vi "Abort Multipart Upload.vi"(8 "error in (no error)":errorcluster, 11 "Multipart Upload RefNum in":T1) -> (0 "error out":errorcluster, 2 "No Such Upload":bool, 3 "Multipart Upload RefNum out":T1)   [LabVIEW 2011, in "LV Interface for Amazon S3.lvlib"]
doc: "This operation <B>aborts a multipart upload</B>. After a multipart upload is aborted, <B>no additional parts can be uploaded using that multipart upload reference</B>. The <B>storage consumed</B> by any previously uploaded parts <B>will be freed</B>. However, <B>if any part uploads are currently in progress, those</B> part uploads <B>might or might not succeed</B>. As a result, <B>it might be necessary to abort a given multipart upload multiple times</B> in order to completely free all storage consumed by all parts."
uses:
  LV Interface for Amazon S3.lvlib
  Typedefs/AMZ_S3_Multipart Upload RefNum.ctl
  Typedefs/AMZ_S3_Multipart Upload RefNum Enum.ctl
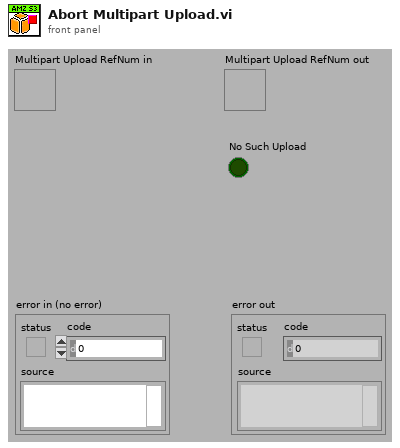
[diagram p1: front panel]
types:
  T1 = typedef "LV Interface for Amazon S3.lvlib/AMZ_S3_Multipart Upload RefNum.ctl" = refnum<k1>
  T2 = typedef "LV Interface for Amazon S3.lvlib/AMZ_S3_Multipart Upload Data.ctl" = cluster{"Object":string, "Bucket":string, "UploadID":string, "Parts":T3[]}
  T3 = typedef "LV Interface for Amazon S3.lvlib/AMZ_S3_Multipart Upload Part Data.ctl" = cluster{"PartNumber":u16, "Lat modified":timestamp, "ETag":string, "Size":u64}
  T4 = typedef "LV Interface for Amazon S3.lvlib/AMZ_S3_Call Results.ctl" = enum16{"Success", "UndefinedError", "AccessDenied", "AccountProblem", "AmbiguousGrantByEmailAddress", "BadDigest", "BucketAlreadyExists", "BucketAlreadyOwnedByYou", "BucketNotEmpty", "CredentialsNotSupported", "CrossLocationLoggingProhibited", "EntityTooSmall", "EntityTooLarge", "ExpiredToken", "IllegalVersioningConfigurationException", "IncompleteBody", "IncorrectNumberOfFilesInPostRequest", "InlineDataTooLarge", "InternalError", "InvalidAccessKeyId", "InvalidAddressingHeader", "InvalidArgument", "InvalidBucketName", "InvalidDigest", "InvalidLocationConstraint", "InvalidPart", "InvalidPartOrder", "InvalidPayer", "InvalidPolicyDocument", "InvalidRange", "InvalidSecurity", "InvalidSOAPRequest", "InvalidStorageClass", "InvalidTargetBucketForLogging", "InvalidToken", "InvalidURI", "KeyTooLong", "MalformedACLError", "MalformedPOSTRequest", "MalformedXML", "MaxMessageLengthExceeded", "MaxPostPreDataLengthExceededError", "MetadataTooLarge", "MethodNotAllowed", "MissingAttachment", "MissingContentLength", "MissingRequestBodyError", "MissingSecurityElement", "MissingSecurityHeader", "NoLoggingStatusForKey", "NoSuchBucket", "NoSuchKey", "NoSuchUpload", "NoSuchVersion", "NotImplemented", "NotSignedUp", "OperationAborted", "PermanentRedirect", "PreconditionFailed", "Redirect", "RequestIsNotMultiPartContent", "RequestTimeout", "RequestTimeTooSkewed", "RequestTorrentOfBucketError", "SignatureDoesNotMatch", "SlowDown", "TemporaryRedirect", "TokenRefreshRequired", "TooManyBuckets", "UnexpectedContent", "UnresolvableGrantByEmailAddress", "UserKeyMustBeSpecified", "LabVIEWError"}
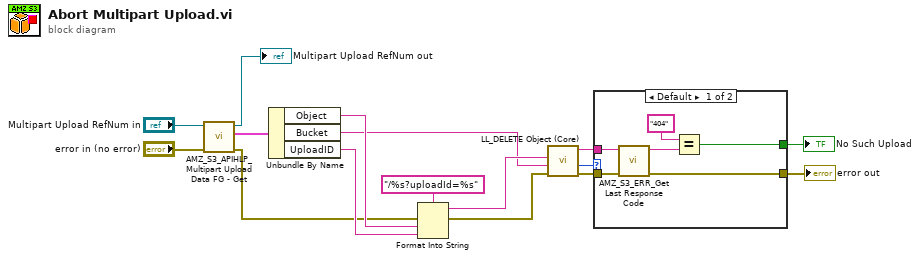
[diagram p0: block diagram]
diagram:
  n1 = call "AMZ_S3_APIHLP_Multipart Upload Data FG - Get.vi"("error in (no error)"="error in (no error)", "Multipart Upload RefNum in"="Multipart Upload RefNum in") -> ("error out"=w3:errorcluster, "Multipart Upload Data"=w11:T2, "Multipart Upload RefNum out"=→"Multipart Upload RefNum out":T1)  [unwired: 7 in]
  n2 = Unbundle By Name(w11) -> ("Object"=w12:string, "Bucket"=w7:string, "UploadID"=w13:string)
  n3 = Format Into String(format string="/%s?uploadId=%s", error in=w3, w12, w13) -> (resulting string=w8:string, error out=w6:errorcluster)  [unwired: 1 in]
  n4 = call "LL_DELETE Object (Core).vi"("error in (no error)"=w6, "Bucket"=w7, "Path and query string"=w8) -> ("error out"=w5:errorcluster, "Call Result"=w1:T4, "Response header"=w4:string)  [unwired: 5 in, 1 out]
  n5 = case shown="Default" w1 {
    tunnel: w5 -> [w22 w23]
    tunnel: w4 -> [w21 _]
    tunnel: [w17 w23] -> w9
    tunnel: [w18 _] -> w2
    frame Default {
      n6 = call "AMZ_S3_ERR_Get Last Response Code.vi"("error in (no error)"=w22, "Response header"=w21) -> ("error out"=w17:errorcluster, "Response code (last)"=w20:string)  [unwired: 8 in]
      n7 = Equal?(x="404", y=w20) -> (x = y?=w18:bool)
    }
    frame "Success" {
    }
  }
  "error out" <- w9
  "No Such Upload" <- w2
